vi "保存计数器功能.vi"(11 "计数器":i32) -> ()   [LabVIEW 2011]
uses:
  Global System.vi
  <vilib>/Utility/config.llb/NI_LVConfig.lvlib
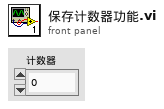
[diagram p1: front panel]
types:
  T1 = typedef "NI_LVConfig.lvlib/Config Data RefNum.ctl" = refnum<k1>
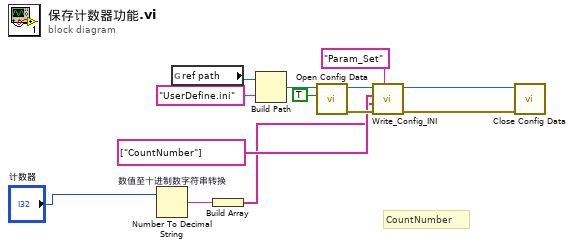
[diagram p0: block diagram]
diagram:
  # "CountNumber"
  n1 = Number To Decimal String "数值至十进制数字符串转换"(number="计数器") -> (decimal integer string=w2:string)  [unwired: 1 in]
  n2 = global read "Global System.vi" "ref path"() -> (w13:path)
  n3 = Build Array(w2) -> (w1:string[])
  n4 = Build Path(base path=w13, name or relative path="UserDefine.ini" ("名称或相对路径")) -> (appended path=w10:path)
  n5 = call <vilib>:"Open Config Data.vi"("create file if necessary (T)"=TRUE, "configuration file path"=w10) -> ("error out"=w8:errorcluster, "refnum"=w9:T1)  [unwired: 7 in, 1 out]
  n6 = call "Write_Config_INI.vi"("section"="Param_Set", "error in (no error)"=w8, "Inputs"=w1, "Keys"=string[] ["CountNumber"], "refnum"=w9) -> ("error out"=w5:errorcluster, "refnum 2"=w6:T1)  [unwired: 5 in]
  n7 = call <vilib>:"Close Config Data.vi"("error in (no error)"=w5, "refnum"=w6) -> ()  [unwired: 8 in, 2 out]
